vi "Do.vi"(8 "error in":errorcluster, 10 "Actor in":refnum<class "Actor.lvclass">, 11 "Update Heater DC MSG":refnum<class "Update Heater DC MSG.lvclass">) -> (0 "error out":errorcluster, 2 "Actor out":refnum<class "Actor.lvclass">)   [LabVIEW 2017, in "Controller.lvlib" / "Update Heater DC MSG.lvclass"]
doc: "(<B>Filename</B>: Actor Framework.lvlib:Message.lvclass:Do.vi)\n\nDefines what a message does when it is received by an actor. Generally, a message instructs an actor to invoke one of its methods. By default, this method does nothing. A child class must override it to define behavior. Create a child class by using the Actor Framework Message Maker dialog box."
uses:
  Update Heater DC MSG.lvclass
  <vilib>/ActorFramework/Actor/Actor.lvclass
  Update Heater DC MSG.lvclass/Update Heater DC MSG.ctl
  gController.lvclass
  C:/Program Files (x86)/National Instruments/LabVIEW 2017/vi.lib/MSR Consulting, LLC/General Reuse/SuperActor/SuperActor.lvclass
  C:/Program Files (x86)/National Instruments/LabVIEW 2017/vi.lib/ActorFramework/Actor/Actor.lvclass
  <vilib>/MSR Consulting, LLC/General Reuse/SuperActor/SuperActor.lvclass/SuperActor.ctl
  <vilib>/MSR Consulting, LLC/General Reuse/SuperActor/Read CVT Session.vi
  <vilib>/MSR Consulting, LLC/General Reuse/SuperActor/Read Log Session.vi
  <vilib>/rvi/errors/niLvFpgaAdjustHostInterfaceError.vi
  <vilib>/Utility/error.llb/Error Cluster From Error Code.vi
  FPGA Ref.ctl
  <vilib>/rvi/interface/nirviReadWriteControl/nirviReadWriteControl.xnode
  FPGA Bitfiles/server_v1_2_1_4.lvbitx
  <vilib>/MSR Consulting, LLC/General Reuse/Session APIs/_Session Fwk/Session - Root.lvclass
  NiFpgaLv.dll
  <vilib>/MSR Consulting, LLC/General Reuse/Session APIs/CVT/CVT.lvclass
  <vilib>/MSR Consulting, LLC/General Reuse/Session APIs/Session Log/System Log.lvclass
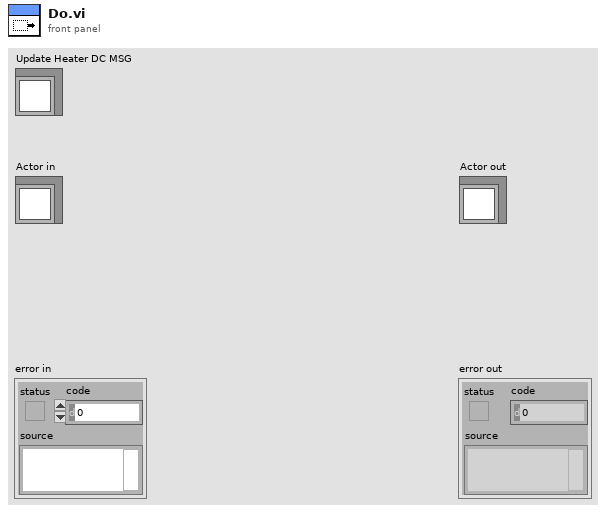
[diagram p1: front panel]
types:
  T1 = typedef "Session - Root.lvclass/Session Handle.ctl" = refnum<data-value>
  T2 = typedef "FPGA Ref.ctl" = refnum<k20>
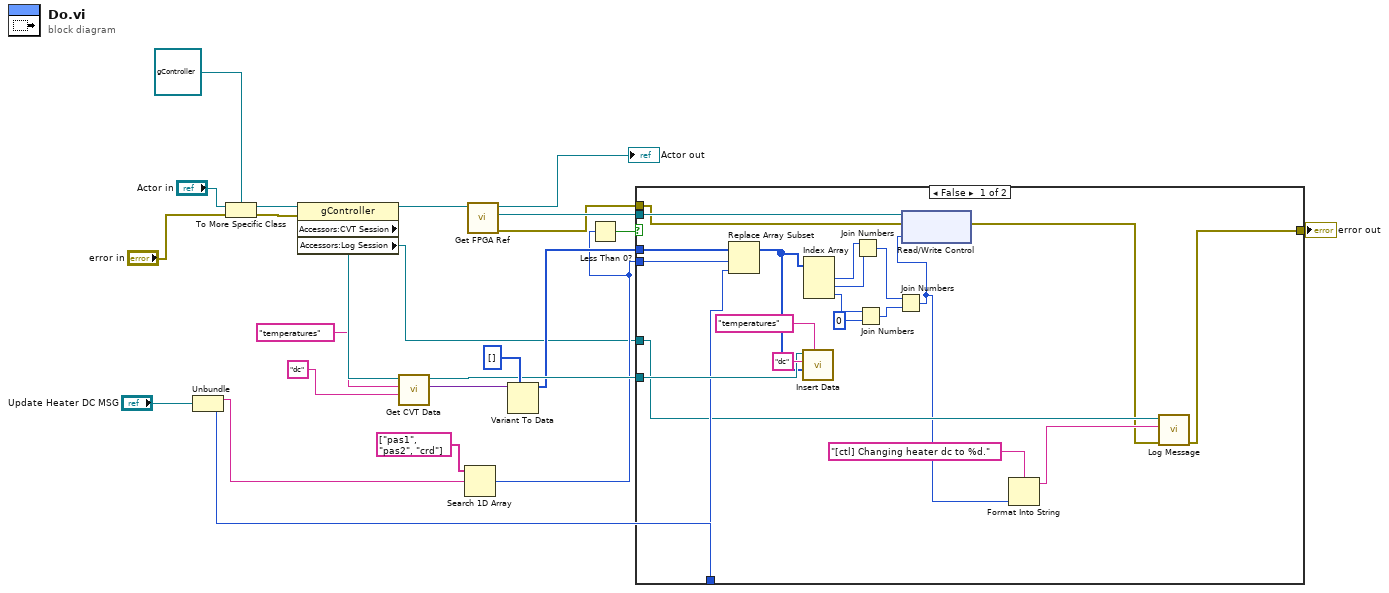
[diagram p0: block diagram]
diagram:
  n1 = Unbundle("Update Heater DC MSG") -> (w9:string, w6:u8)
  n2 = To More Specific Class(target class=refnum<class "gController.lvclass"> refnum ("Controller.lvlib:gController"), reference="Actor in", error in="error in") -> (specific class reference=w18:refnum<class "gController.lvclass">, error out=w17:errorcluster)
  n3 = property class="gController"(reference=w18, error in=w17) -> (reference out=w16:refnum<class "gController.lvclass">, "Accessors:CVT Session"=w15:T1, "Accessors:Log Session"=w1:T1)  [unwired: 1 out]
  n4 = call <vilib>:"Get CVT Data.vi"("Variable"="dc" ("tag"), "Group"="temperatures", "CVT Session In"=w15) -> ("Data Out"=w12:variant, "CVT Session Out"=w8:T1)  [unwired: 5 in, 2 out]
  n5 = Search 1D Array(1D array=string[] ["pas1", "pas2", "crd"], element=w9) -> (index of element=w4:i32)  [unwired: 1 in]
  n6 = call "Get FPGA Ref.vi"("Actor In"=w16) -> ("error out"=w2:errorcluster, "FPGA Ref"=w20:T2, "Actor Out"=→"Actor out":refnum<class "Actor.lvclass">)  [unwired: 8 in]
  n7 = Variant To Data(type=u8[] [], Variant=w12) -> (data=w7:u8[])  [unwired: 1 in, 1 out]
  n8 = Less Than 0?(x=w4) -> (x < 0?=w5:bool)
  n9 = case shown="False" w5 {
    tunnel: w20 -> [w45 _]
    tunnel: w8 -> [w42 _]
    tunnel: w7 -> [w41 _]
    tunnel: w6 -> [w40 _]
    tunnel: w4 -> [w39 _]
    tunnel: [w25 w46] -> w3
    tunnel: w2 -> [w31 w46]
    tunnel: w1 -> [w30 _]
    frame False {
      n10 = Replace Array Subset(array=w41, new element=w40, index=w39) -> (w38:u8[])
      n11 = call <vilib>:"Insert Data.vi"("Group"="temperatures", "Data"=w38, "tag"="dc", "CVT Session In"=w42) -> ()  [unwired: 6 in, 2 out]
      n12 = Index Array(array=w38) -> (element #1=w37:u8, element #2=w36:u8, element #3=w35:u8)  [unwired: 3 in]
      n13 = Join Numbers(hi=w37, lo=w36) -> ((hi.lo)=w33:u16)
      n14 = Join Numbers(hi=w35, lo=u8 0) -> ((hi.lo)=w32:u16)
      n15 = Join Numbers(hi=w33, lo=w32) -> ((hi.lo)=w29:u32)
      n16 = xnode "Read/Write Control"("FPGA VI Reference In"=w45, "error in"=w31, "HeaterDC"=w29) -> ("error out"=w26:errorcluster)  [unwired: 1 out]
      n17 = Format Into String(format string="[ctl] Changing heater dc to %d.", w29) -> (resulting string=w27:string)  [unwired: 2 in, 1 out]
      n18 = call <vilib>:"Log Message.vi"("error in"=w26, "MSG In"=w27, "session in"=w30) -> ("error out"=w25:errorcluster)  [unwired: 7 in, 1 out]
    }
    frame True {
    }
  }
  "error out" <- w3
